vi "setChannel.vi"(8 "error in (no error)":errorcluster, 10 "channel":i32, 11 "Radio in":refnum<class "Radio.lvclass">) -> (0 "error out":errorcluster, 3 "Radio out":refnum<class "Radio.lvclass">)   [LabVIEW 2018, in "Radio.lvclass"]
uses:
  Radio.lvclass
  Device Class/Device.lvclass
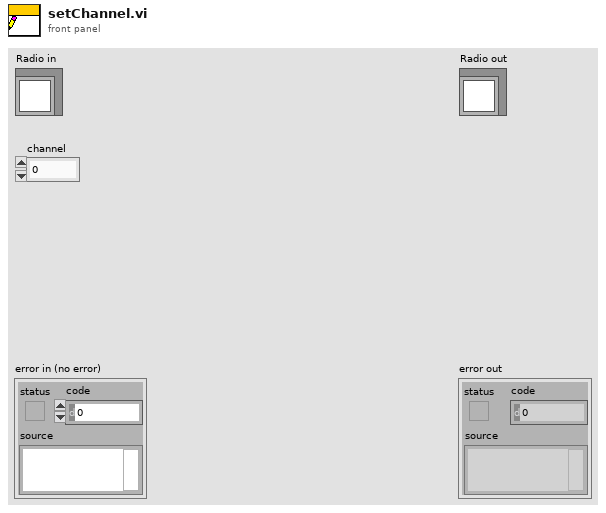
[diagram p1: front panel]
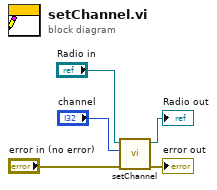
[diagram p0: block diagram]
diagram:
  n1 = call-parent "setChannel.vi"("error in (no error)"="error in (no error)", "channel"="channel", "Device in"="Radio in") -> ("error out"=→"error out":errorcluster, "Device out"=→"Radio out":refnum<class "Radio.lvclass">)  [unwired: 7 in]
